vi "F Dwf Digital Uart Rx.vi"(0 "hdwf":i32, 1 "pParity":i32, 5 "szRx":string, 7 "cRx":i32, 9 "pcRx":i32, 11 "error in (no error)":errorcluster) -> (3 "pParity out":i32, 4 "function return":i32, 6 "szRx out":string, 10 "pcRx out":i32, 15 "error out":errorcluster)   [LabVIEW 2021, in "Olasdwf.lvlib"]
doc: "DWFAPI int FDwfDigitalUartRx(HDWF hdwf, char *szRx, int cRx, int *pcRx, int *pParity);"
uses:
  Olasdwf.lvlib
  Windows/System32/dwf.dll
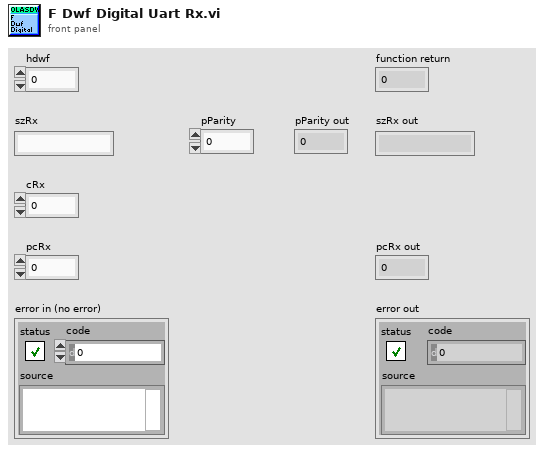
[diagram p1: front panel]
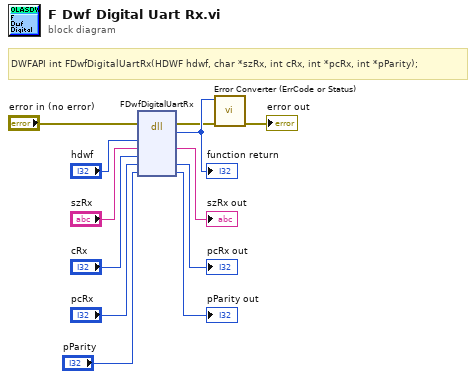
[diagram p0: block diagram]
diagram:
  # "DWFAPI int FDwfDigitalUartRx(HDWF hdwf, char *szRx, int cRx, int *pcRx, int *pParity);"
  n1 = dll-call lib="/Windows/System32/dwf.*" fn="FDwfDigitalUartRx"(error in="error in (no error)", "hdwf"="hdwf", "szRx"="szRx", "cRx"="cRx", "pcRx"="pcRx", "pParity"="pParity") -> (error out=w2:errorcluster, w12:i32, "szRx"=→"szRx out":string, "pcRx"=→"pcRx out":i32, "pParity"=→"pParity out":i32)  [unwired: 4 in, 1 out]
  "function return" <- w12
  n2 = call "Error Converter (ErrCode or Status).vi"("error in (no error)"=w2, "error code"=w12) -> ("error out"=→"error out":errorcluster)  [unwired: 9 in]
